vi "index values of B.vi"() -> ()   [LabVIEW 2022 SP3]
panel:
  in  "index values of B":i32[](array[numeric])
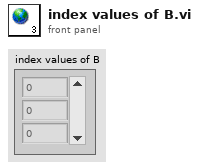
[diagram p1: front panel]
diagram:
